vi "IsAnyOfType.vi"(8 "error in":errorcluster, 9 "Message Type":string, 10 "Any":T1, 11 "gRPCid in":T2) -> (0 "error out":errorcluster, 1 "Is Type":bool, 3 "gRPCid out":T2)   [LabVIEW 2019, in "grpc-lvsupport.lvlib"]
uses:
  grpc-lvsupport.lvlib
  grpcId.ctl
  Any.ctl
  <resource>/libgrpc_labview.dll
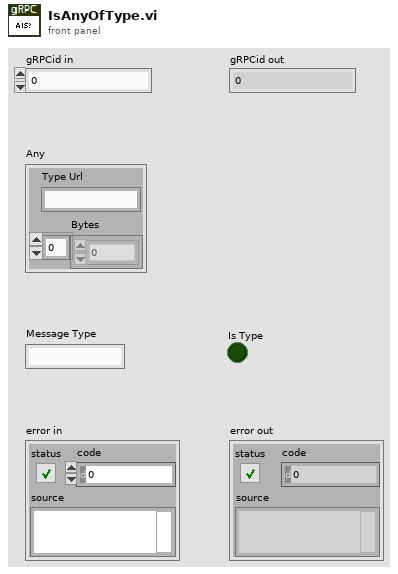
[diagram p1: front panel]
types:
  T1 = typedef "grpc-lvsupport.lvlib/Any.ctl" = cluster{"Type Url":string, "Bytes":u8[]}
  T2 = typedef "grpc-lvsupport.lvlib/grpcId.ctl" = u64
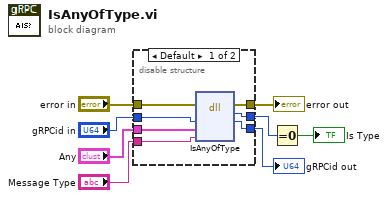
[diagram p0: block diagram]
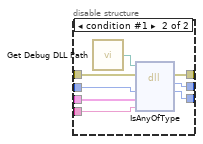
[diagram p2: hidden frame]
diagram:
  n1 = disable-structure shown="Default" {
    disable-tunnel: "error in" -> [w15 w23]
    disable-tunnel: [w14 w22] -> w7
    disable-tunnel: "gRPCid in" -> [w13 w20]
    disable-tunnel: [w12 w19] -> w5
    disable-tunnel: "Message Type" -> [w11 w18]
    disable-tunnel: [w10 w17] -> w3
    disable-tunnel: "Any" -> [w9 w16]
    frame condition #0 (active) {
      n2 = dll-call lib="C:/Program Files (x86)/National Instruments/LabVIEW 2024/resource/libgrpc_labview.*" fn="IsAnyOfType"(error in=w15, "gRPCId"=w13, "any"=w9, "messageType"=w11) -> (error out=w14:errorcluster, "return type"=w10:i32, "gRPCId"=w12:u64)  [unwired: 4 in, 1 out]
    }
    frame condition #1 {
      n3 = call "Get Debug DLL Path.vi"() -> ("DLL Path"=w21:path)
      n4 = dll-call lib="?" fn="IsAnyOfType"(path in=w21, error in=w23, "gRPCId"=w20, "any"=w16, "messageType"=w18) -> (error out=w22:errorcluster, "return type"=w17:i32, "gRPCId"=w19:u64)  [unwired: 3 in, 1 out]
    }
  }
  "gRPCid out" <- w5
  "error out" <- w7
  n5 = Equal To 0?(x=w3) -> (x = 0?=→"Is Type":bool)
